vi "CreateTableDbUnderstanding.vi"() -> ()   [LabVIEW 2019]
uses:
  <vilib>/addons/database/Auxilliary.llb/DB Tools Column Info.ctl
  <vilib>/addons/database/Auxilliary.llb/DB Tools DataTypes.ctl
  <vilib>/addons/database/Connection.llb/DB Tools Open Connec (String).vi
  <vilib>/addons/database/NI_Database_API.lvlib
panel:
  in  "Connection Information ( Provide your ODBC Server Name Here )":string
  in  "Table Name":string
  out "error out":errorcluster
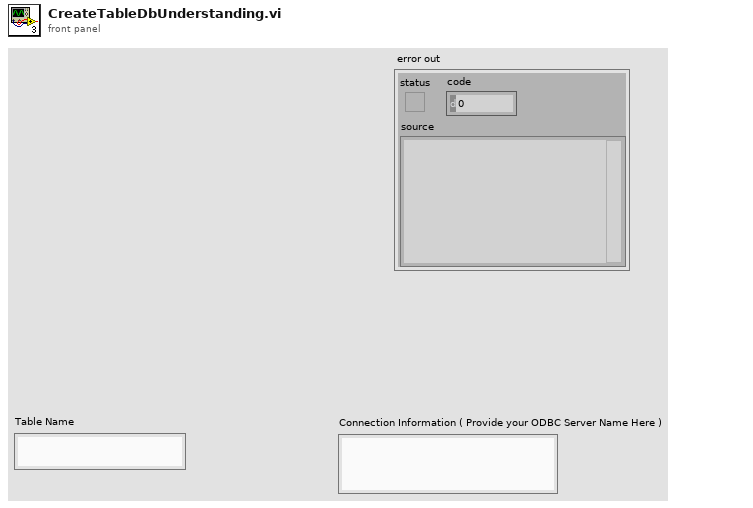
[diagram p1: front panel]
types:
  T1 = typedef "NI_Database_API.lvlib/DB Tools Column Info.ctl" = cluster{"column name":string, "data type":T2, "size":i32, "allow null?":bool}
  T2 = typedef "NI_Database_API.lvlib/DB Tools DataTypes.ctl" = enum16{"String", "Long (I32)", "Single (SGL)", "Double (DBL)", "Date/Time", "Binary"}
  T3 = typedef "NI_Database_API.lvlib/Conn ObjectReference.ctl" = refnum<k1>
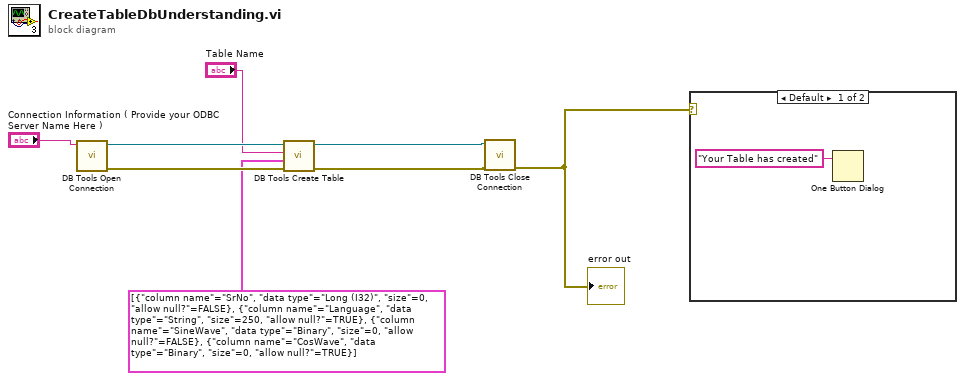
[diagram p0: block diagram]
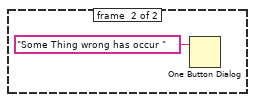
[diagram p2: hidden frame]
diagram:
  n1 = call-poly <vilib>:"DB Tools Open Connection.vi"("connection information"="Connection Information ( Provide your ODBC Server Name Here )") -> ("error out"=w7:errorcluster, "connection reference"=w8:T3)  [unwired: 7 in]
  n2 = call <vilib>:"DB Tools Create Table.vi"("error in (no error)"=w7, "column information"=T1[] [{"column name"="SrNo", "data type"=enum."Long (I32)", "size"=0, "allow null?"=FALSE}, {"column name"="Language", "data type"=enum."String", "size"=250, "allow null?"=TRUE}, {"column name"="SineWave", "data type"=enum."Binary", "size"=0, "allow null?"=FALSE}, {"column name"="CosWave", "data type"=enum."Binary", "size"=0, "allow null?"=TRUE}], "table"="Table Name", "connection reference"=w8) -> ("error out"=w5:errorcluster, "connection reference out"=w6:T3)  [unwired: 4 in]
  n3 = call <vilib>:"DB Tools Close Connection.vi"("error in (no error)"=w5, "connection reference"=w6) -> ("error out"=w1:errorcluster)  [unwired: 5 in]
  "error out" <- w1
  n4 = case shown="Default" w1 {
    frame #0 {
      n5 = One Button Dialog(message="Your Table has created") -> ()  [unwired: 1 in, 1 out]
    }
    frame #1 {
      n6 = One Button Dialog(message="Some Thing wrong has occur ") -> ()  [unwired: 1 in, 1 out]
    }
  }
